vi "Test Switch Tables 2.vi"() -> ()   [LabVIEW 2019, in "LV-Data.PGSQL.lvclass"]
uses:
  LV-Data.PGSQL.lvclass
  <vilib>/addons/_JKI Toolkits/Caraya/classes/Assert/Assert Not Error.vi
  <vilib>/addons/_JKI Toolkits/Caraya/classes/Test/Test.lvclass
  <vilib>/addons/_JKI Toolkits/Caraya/classes/Assert/Assert.lvclass
panel:
  out "error out":errorcluster
  in  "error in (no error)":errorcluster
  out "Data.PG out":refnum<class "LV-Data.PGSQL.lvclass">
  in  "Data.PG":refnum<class "LV-Data.PGSQL.lvclass">
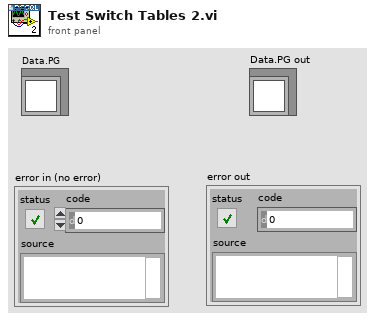
[diagram p1: front panel]
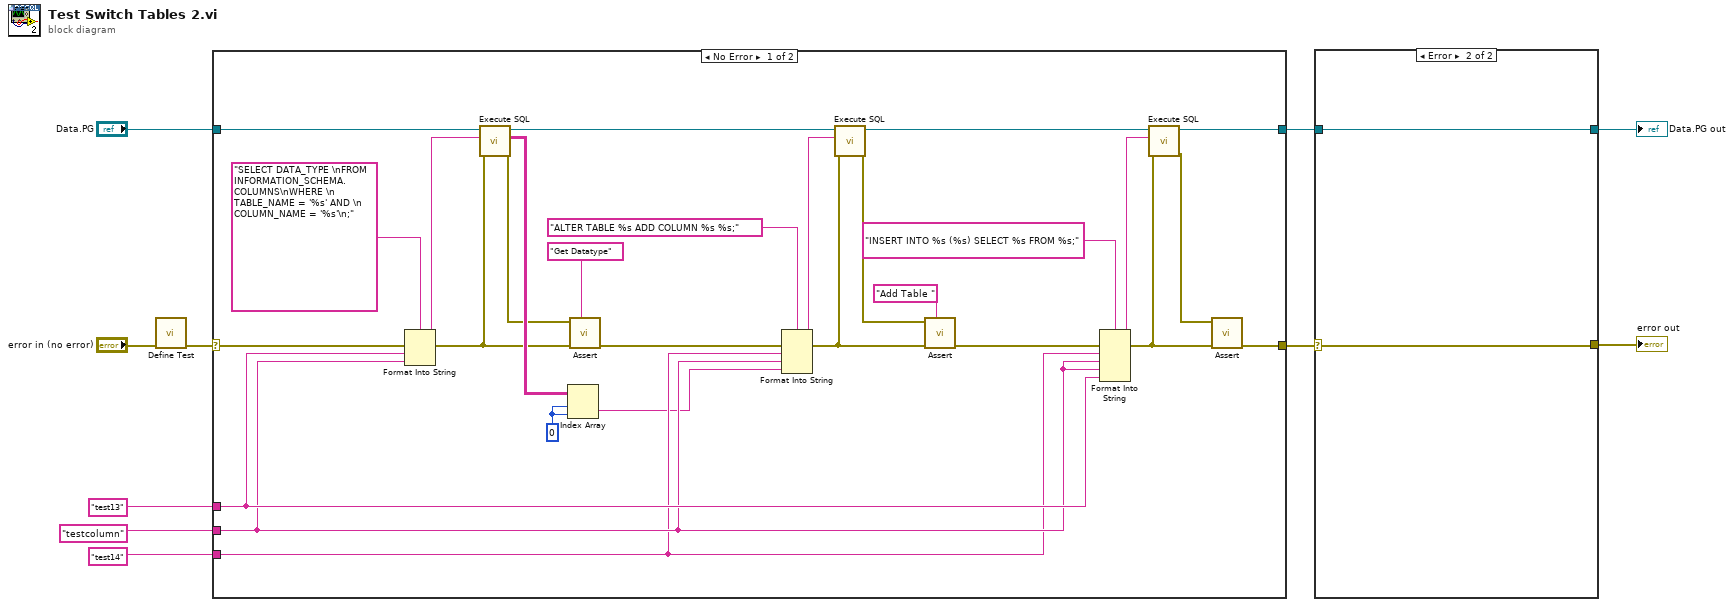
[diagram p0: block diagram]
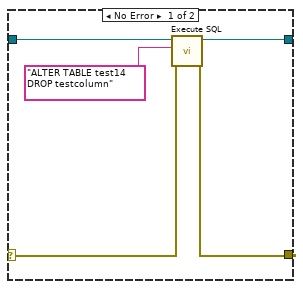
[diagram p3: hidden frame]
diagram:
  n1 = call <vilib>:"Define Test.vi"("error in (no error)"="error in (no error)") -> ("error out"=w2:errorcluster)  [unwired: 10 in]
  n2 = case shown="No Error" w2 {
    selector: w2 -> [w23 w39]
    tunnel: "test14" ("Old Column") -> [w25 _]
    tunnel: "testcolumn" ("Old Column") -> [w26 _]
    tunnel: "Data.PG" -> [w24 w40]
    tunnel: [w38 w40] -> w4
    tunnel: "test13" ("Old Table") -> [w27 _]
    tunnel: [w16 w39] -> w3
    frame No Error {
      w31 = 0 ("index (row)")
      n3 = Format Into String(format string="SELECT DATA_TYPE \nFROM INFORMATION_SCHEMA.COLUMNS\nWHERE \n     TABLE_NAME = '%s' AND \n     COLUMN_NAME = '%s'\n;", error in=w23, w27, w26) -> (resulting string=w28:string, error out=w13:errorcluster)  [unwired: 1 in]
      n4 = call "Execute SQL.vi"("error in"=w13, "SQL"=w28, "LV-Data.PGSQL"=w24) -> ("error out"=w12:errorcluster, "Result"=w37:string[][], "LV-Data.PGSQL out"=w33:refnum<class "LV-Data.PGSQL.lvclass">)  [unwired: 6 in]
      n5 = Index Array(array=w37, index (row)=w31, index (col)=w31) -> (element=w11:string)
      n6 = call-poly <vilib>:"Assert.vi"("Label"="Get Datatype", "error in (no error)"=w13, "Not Error?"=w12) -> ("error out"=w22:errorcluster)  [unwired: 8 in]
      n7 = Format Into String(format string="ALTER TABLE %s ADD COLUMN %s %s;", error in=w22, w25, w26, w11) -> (resulting string=w34:string, error out=w14:errorcluster)  [unwired: 1 in]
      n8 = call "Execute SQL.vi"("error in"=w14, "SQL"=w34, "LV-Data.PGSQL"=w33) -> ("error out"=w19:errorcluster, "LV-Data.PGSQL out"=w32:refnum<class "LV-Data.PGSQL.lvclass">)  [unwired: 6 in, 1 out]
      n9 = call-poly <vilib>:"Assert.vi"("Label"="Add Table ", "error in (no error)"=w14, "Not Error?"=w19) -> ("error out"=w20:errorcluster)  [unwired: 8 in]
      n10 = Format Into String(format string="INSERT INTO %s (%s) SELECT %s FROM %s;", error in=w20, w25, w26, w26, w27) -> (resulting string=w29:string, error out=w15:errorcluster)  [unwired: 1 in]
      n11 = call "Execute SQL.vi"("error in"=w15, "SQL"=w29, "LV-Data.PGSQL"=w32) -> ("error out"=w17:errorcluster, "LV-Data.PGSQL out"=w38:refnum<class "LV-Data.PGSQL.lvclass">)  [unwired: 6 in, 1 out]
      n12 = call-poly <vilib>:"Assert.vi"("error in (no error)"=w15, "Not Error?"=w17) -> ("error out"=w16:errorcluster)  [unwired: 9 in]
    }
    frame Error {
    }
  }
  n13 = case shown="Error" w3 {
    selector: w3 -> [w41 w47]
    tunnel: [w44 w47] -> w6
    tunnel: [w45 w46] -> w5
    tunnel: w4 -> [w42 w46]
    frame No Error {
      n14 = call "Execute SQL.vi"("error in"=w41, "SQL"="ALTER TABLE test14 DROP testcolumn", "LV-Data.PGSQL"=w42) -> ("error out"=w44:errorcluster, "LV-Data.PGSQL out"=w45:refnum<class "LV-Data.PGSQL.lvclass">)  [unwired: 6 in, 1 out]
    }
    frame Error {
    }
  }
  "Data.PG out" <- w5
  "error out" <- w6
